vi "Interpolator port.vi"(8 "Current Distance (ft)":dbl=141.0 format="%0.2f", 11 "Interpolation Table":dbl[][](array[numeric])=[[60.0, 133.0, 177.0, 222.0]] format="%0.2f") -> (3 "Corrected DIstance":dbl=133.0 format="%0.2f")   [LabVIEW 2019]
uses:
  <vilib>/Analysis/NI_AALPro.lvlib
panel:
  # "We train these values when we set up the shooter. We can also add these to the dashboard so we can tweak them. This will make setting up our shooter simple and easy to adjust."
  # "We output this number to the PID loop to control the speed of the shooter."
  # "We get the distance from the vision software and feed it into the interpolator."
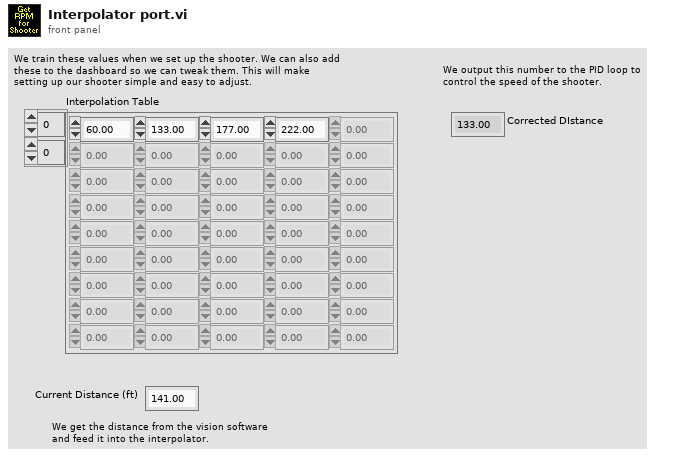
[diagram p1: front panel]
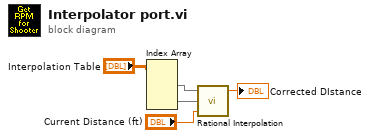
[diagram p0: block diagram]
diagram:
  n1 = Index Array(array="Interpolation Table") -> (element #1=w2:dbl[], element #2=w1:dbl[])  [unwired: 4 in]
  n2 = call <vilib>:"Rational Interpolation.vi"("x value"="Current Distance (ft)", "X"=w1, "Y"=w2) -> ("interpolation value"=→"Corrected DIstance":dbl)  [unwired: 2 out]
